vi "hardware_initialize_hardware.vi"(8 "error in (no error)":errorcluster, 11 "hydraharp in":refnum<class "picoharp.lvclass">) -> (0 "error out":errorcluster, 3 "hydraharp out":refnum<class "picoharp.lvclass">)   [LabVIEW 2015, in "picoharp.lvclass"]
uses:
  picoharp.lvclass
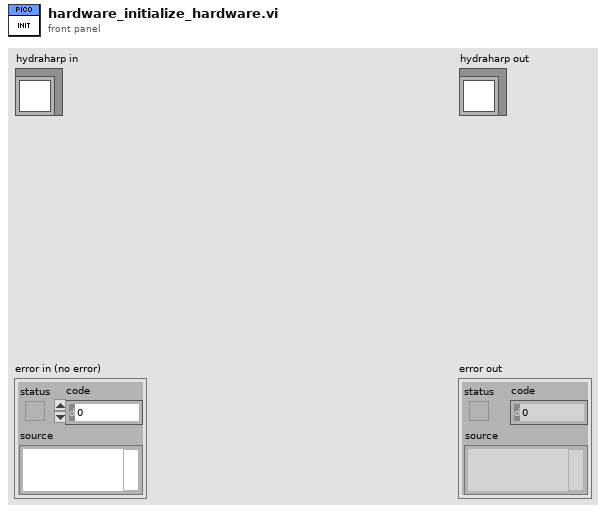
[diagram p1: front panel]
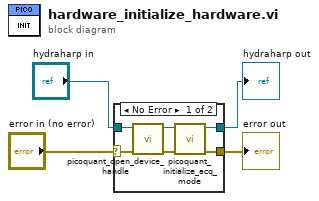
[diagram p0: block diagram]
diagram:
  n1 = case shown="No Error" "error in (no error)" {
    selector: "error in (no error)" -> [w7 w11]
    tunnel: "hydraharp in" -> [w8 w12]
    tunnel: [w5 w11] -> w2
    tunnel: [w6 w12] -> w1
    frame No Error {
      n2 = call-dynamic "picoquant_open_device_handle.vi"("error in (no error)"=w7, "picoharp in"=w8) -> ("error out"=w9:errorcluster, "picoharp out"=w10:refnum<class "picoharp.lvclass">)  [unwired: 8 in]
      n3 = call-dynamic "picoquant_initialize_acq_mode.vi"("error in (no error)"=w9, "picoharp in"=w10) -> ("error out"=w5:errorcluster, "picoharp out"=w6:refnum<class "picoharp.lvclass">)  [unwired: 8 in]
    }
    frame Error {
    }
  }
  "error out" <- w2
  "hydraharp out" <- w1
